vi "Zähler_reset_FGV.vi"(0 "Band/Station Index":T2, 1 "Modus":T1(ring), 3 "gewünschter Zählerwert":u16, 4 "Zähler":enum16{"Zähler 1", "Zähler 2", "Zähler 3"}(ring)) -> (5 "Zählerwerte":u16[](array[numeric]), 6 "zurücksetzen":bool[](array[boolean]), 7 "Werte verändert":bool)   [LabVIEW 2013, in "cRIO_FPGA_COMMUNICATION.lvlib"]
uses:
  TYPES/TYPE Station Index.ctl
  cRIO_FPGA_COMMUNICATION.lvlib
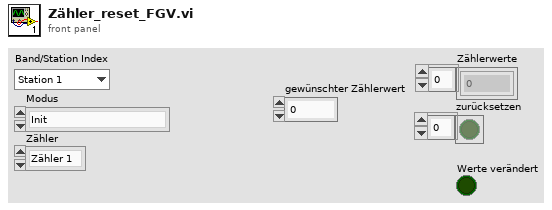
[diagram p1: front panel]
types:
  T1 = enum16{"Init", "Zählerwert nullen", "Zählerwert setzen", "lese gesetzten Zählerwert"}
  T2 = typedef "cRIO_FPGA_COMMUNICATION.lvlib/TYPE Station Index.ctl" = enum16{"Station 1", "Station 2", "Station 3", "Station 4", "Station 5", "Station 6", "Station 7", "Station 8", "Station 9", "Station 10", "Station 11", "Station 12", "Station 13", "Station 14", "Station 15", "Station 16", "Station 17", "Station 18", "Station 19", "Station 20"}
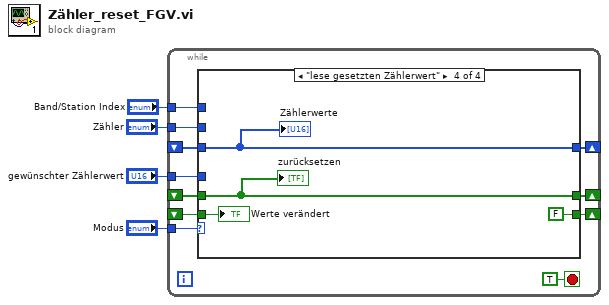
[diagram p0: block diagram]
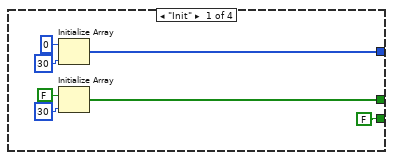
[diagram p2: hidden frame]
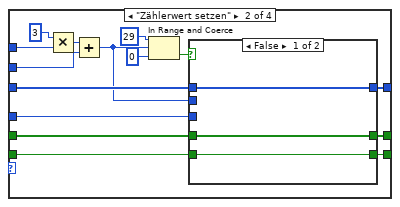
[diagram p3: hidden frame]
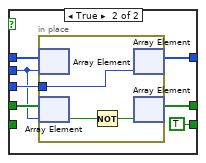
[diagram p4: hidden frame]
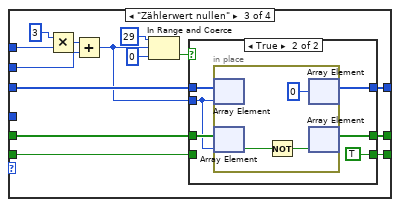
[diagram p5: hidden frame]
diagram:
  n1 = while {
    tunnel: "Modus" -> [w14]
    tunnel: "gewünschter Zählerwert" -> [w13]
    tunnel: "Band/Station Index" -> [w12]
    tunnel: "Zähler" -> [w11]
    shift-right: [w10] -> _
    shift-left: _ -> [w9]
    shift-right: [w8] -> _
    shift-left: _ -> [w7]
    shift-right: [w6] -> _
    shift-left: _ -> [w5]
    stop <- TRUE stop-if-true
    n2 = case shown="\"lese gesetzten Zählerwert\"" w14 {
      tunnel: w13 -> [_ w29 _ _]
      tunnel: w12 -> [_ w35 w62 _]
      tunnel: w11 -> [_ w34 w61 _]
      tunnel: [w21 w32 w59 w79] -> w10
      tunnel: w9 -> [_ w33 w60 w79]
      tunnel: [w18 w30 w57 w80] -> w8
      tunnel: w7 -> [_ w31 w58 w80]
      tunnel: [FALSE w24 w52 FALSE] -> w6
      tunnel: w5 -> [_ w23 w51 w78]
      frame "Init" {
        n3 = Initialize Array(u16 0 ("Dimension"), 30 ("Dimension")) -> (w18:u16[])
        n4 = Initialize Array(FALSE, 30 ("Dimension")) -> (w21:bool[])
      }
      frame "Zählerwert setzen" {
        n5 = Multiply(x=3, y=w35) -> (x*y=w37:i32)
        n6 = Add(x=w37, y=w34) -> (x+y=w25:i32)
        n7 = In Range and Coerce(upper limit=29 ("Obergrenze"), x=w25, lower limit=0 ("Untergrenze")) -> (In Range?=w26:bool)  [unwired: 1 out]
        n8 = case shown="False" w26 {
          tunnel: w33 -> [w39 w47]
          tunnel: [w39 w46] -> w32
          tunnel: w31 -> [w40 w45]
          tunnel: [w40 w44] -> w30
          tunnel: w29 -> [_ w43]
          tunnel: w25 -> [_ w42]
          tunnel: [w38 TRUE] -> w24
          tunnel: w23 -> [w38 _]
          frame False {
          }
          frame True {
            n9 = in-place {
              in-place-border: w43 -> [w48]
              n10 = in-place-array #1(w45, w42) -> ()  [unwired: 1 out]
              n11 = in-place-array #2(w47, w42) -> (w50:bool)
              n12 = Not(x=w50) -> (.not. x?=w49:bool)
              n13 = in-place-array #1(w48) -> (w44:u16[])  [unwired: 1 out]
              n14 = in-place-array #2(w49) -> (w46:bool[])  [unwired: 1 out]
            }
          }
        }
      }
      frame "Zählerwert nullen" {
        n15 = Multiply(x=3, y=w62) -> (x*y=w64:i32)
        n16 = Add(x=w64, y=w61) -> (x+y=w53:i32)
        n17 = In Range and Coerce(upper limit=29 ("Obergrenze"), x=w53, lower limit=0 ("Untergrenze")) -> (In Range?=w54:bool)  [unwired: 1 out]
        n18 = case shown="True" w54 {
          tunnel: w60 -> [w66 w73]
          tunnel: [w66 w72] -> w59
          tunnel: w58 -> [w67 w71]
          tunnel: [w67 w70] -> w57
          tunnel: w53 -> [_ w69]
          tunnel: [w65 TRUE] -> w52
          tunnel: w51 -> [w65 _]
          frame False {
          }
          frame True {
            n19 = in-place {
              n20 = in-place-array #3(w71, w69) -> ()  [unwired: 1 out]
              n21 = in-place-array #4(w73, w69) -> (w76:bool)
              n22 = Not(x=w76) -> (.not. x?=w75:bool)
              n23 = in-place-array #3(u16 0 ("Element")) -> (w70:u16[])  [unwired: 1 out]
              n24 = in-place-array #4(w75) -> (w72:bool[])  [unwired: 1 out]
            }
          }
        }
      }
      frame "lese gesetzten Zählerwert" {
        "Zählerwerte" <- w80
        "zurücksetzen" <- w79
        "Werte verändert" <- w78
      }
    }
  }
